vi "disk_tryDeleteFile.vi"(8 "error in (no error)":errorcluster, 11 "path":path) -> (0 "error out":errorcluster)   [LabVIEW 2017, in "NI_ExcelFile.lvlib"]
uses:
  <vilib>/express/express shared/NI_ExcelFile/NI_ExcelFile.lvlib
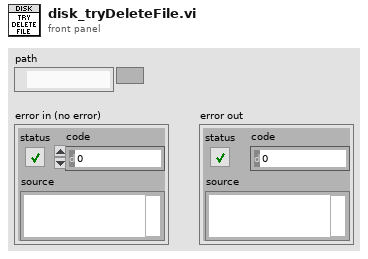
[diagram p1: front panel]
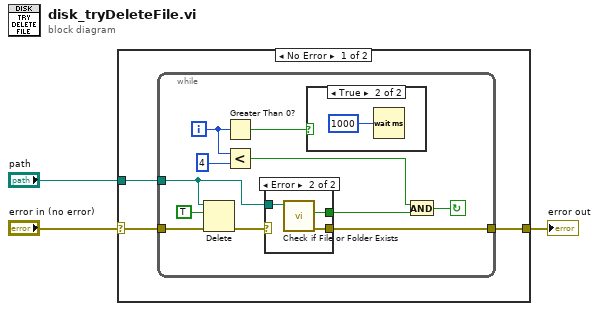
[diagram p0: block diagram]
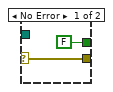
[diagram p3: hidden frame]
diagram:
  n1 = case shown="No Error" "error in (no error)" {
    selector: "error in (no error)" -> [w4 w24]
    tunnel: [w6 w24] -> w3
    tunnel: "path" -> [w5 _]
    frame No Error {
      n2 = while {
        tunnel: w5 -> [w14]
        tunnel: w4 -> [w17]
        tunnel: [w12] -> w6
        i -> [w8]
        stop <- w11 continue-if-true
        n3 = Delete(path (use dialog)=w14, entire hierarchy (F)=TRUE, error in=w17) -> (error out=w15:errorcluster)  [unwired: 2 in, 2 out]
        n4 = Greater Than 0?(x=w8) -> (x > 0?=w7:bool)
        n5 = Less?(x=w8, y=4) -> (x < y?=w9:bool)
        n6 = case shown="Error" w15 {
          selector: w15 -> [w19 _]
          tunnel: w14 -> [_ w23]
          tunnel: [FALSE ("file or folder exists?") w22] -> w10
          tunnel: [w19 w21] -> w12
          frame No Error {
          }
          frame Error {
            n7 = call <vilib>:"Check if File or Folder Exists.vi"("path"=w23) -> ("error out"=w21:errorcluster, "file or folder exists?"=w22:bool)  [unwired: 8 in, 1 out]
          }
        }
        n8 = case shown="True" w7 {
          frame False {
          }
          frame True {
            n9 = Wait (ms)(milliseconds to wait=u32 1000) -> ()  [unwired: 1 out]
          }
        }
        n10 = And(x=w9, y=w10) -> (x .and. y?=w11:bool)
      }
    }
    frame Error {
    }
  }
  "error out" <- w3
